vi "Get Upper-Case.vi"(11 "Letter in":refnum<class "Letter.lvclass">) -> (2 "letter":string, 3 "Letter out":refnum<class "Letter.lvclass">)   [LabVIEW 2015, in "Letter.lvclass"]
uses:
  Letter.lvclass
  Letter.lvclass/Letter.ctl
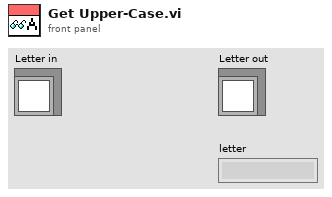
[diagram p1: front panel]
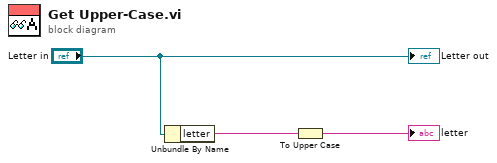
[diagram p0: block diagram]
diagram:
  n1 = Unbundle By Name("Letter in") -> ("letter"=w2:string)
  n2 = To Upper Case(1:w2) -> (0:→"letter":string)
  "Letter out" <- "Letter in"
